vi "LED_Source_Ref-Offset.vi"(0 "Source Resource In":refnum<k15>, 5 "Source channel name":string, 7 "Aperture time":dbl, 9 "LED Voltage (Vo)":dbl, 11 "error in":errorcluster) -> (4 "Source Resource Out":refnum<k15>, 15 "error out":errorcluster)   [LabVIEW 2021, in "start-up.lvlib"]
uses:
  start-up.lvlib
  <instrlib>/niDCPower/nidcpower.llb/niDCPower Source Mode.ctl
  <instrlib>/niDCPower/nidcpower.llb/niDCPower Output Function.ctl
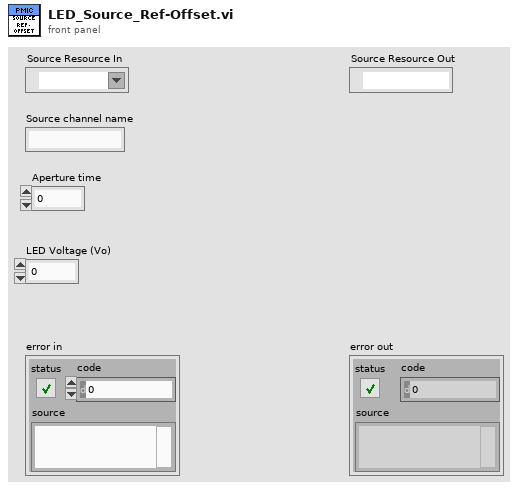
[diagram p1: front panel]
types:
  T1 = typedef "niDCPower Output Function.ctl" = i32
  T2 = typedef "niDCPower Source Mode.ctl" = i32
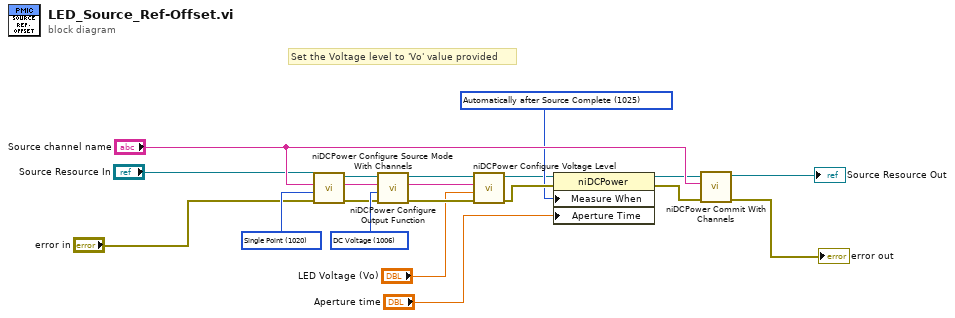
[diagram p0: block diagram]
diagram:
  w12 = T1 1006 items=["DC Voltage"=1006, "DC Current"=1007, "Pulse Voltage"=1049, "Pulse Current"=1050] ("output function")
  w15 = T2 1020 items=["Single Point"=1020, "Sequence"=1021] ("source mode")
  w6 = 1025 items=["Automatically after Source Complete"=1025, "On Demand"=1026, "On Measure Trigger"=1027] ("Measurement:Advanced:Measure When")
  # "Set the Voltage level to 'Vo' value provided"
  n1 = call <instrlib>:"niDCPower Configure Source Mode With Channels.vi"("source mode"=w15, "channel name"="Source channel name", "instrument handle"="Source Resource In") -> ("error out"=w11:errorcluster, "instrument handle out"=w10:refnum<k15>)  [unwired: 7 in]
  n2 = call <instrlib>:"niDCPower Configure Output Function.vi"("error in (no error)"=w11, "output function"=w12, "channel name"="Source channel name", "instrument handle"=w10) -> ("instrument handle out"=w14:refnum<k15>)  [unwired: 7 out]
  n3 = call <instrlib>:"niDCPower Configure Voltage Level.vi"("error in (no error)"="error in", "voltage level"="LED Voltage (Vo)", "channel name"="Source channel name", "instrument handle"=w14) -> ("error out"=w7:errorcluster, "instrument handle out"=w5:refnum<k15>)  [unwired: 6 in]
  n4 = property class="niDCPower"(reference=w5, error in=w7, "Measure When"=w6, "Aperture Time"="Aperture time") -> (reference out=w4:refnum<k15>, error out=w3:errorcluster)
  n5 = call <instrlib>:"niDCPower Commit With Channels.vi"("error in (no error)"=w3, "channel name"="Source channel name", "instrument handle"=w4) -> ("error out"=→"error out":errorcluster, "instrument handle out"=→"Source Resource Out":refnum<k15>)  [unwired: 7 in]
